vi "Position Space Bar Key.vi"(8 "error in (no error)":errorcluster, 10 "z Key":refnum<vi>, 11 "Space bar Key":refnum<vi>) -> (0 "error out":errorcluster)   [LabVIEW 2014]
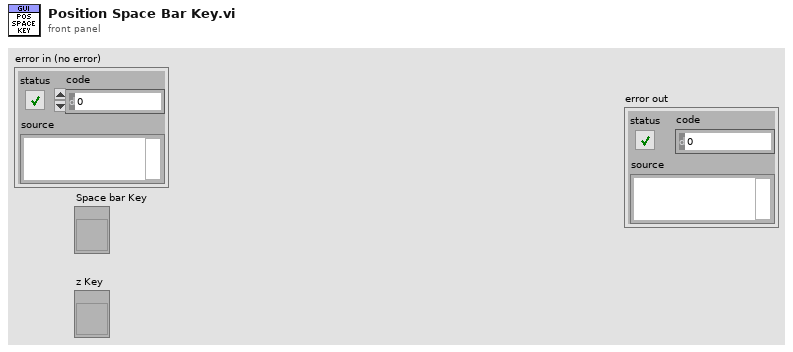
[diagram p1: front panel]
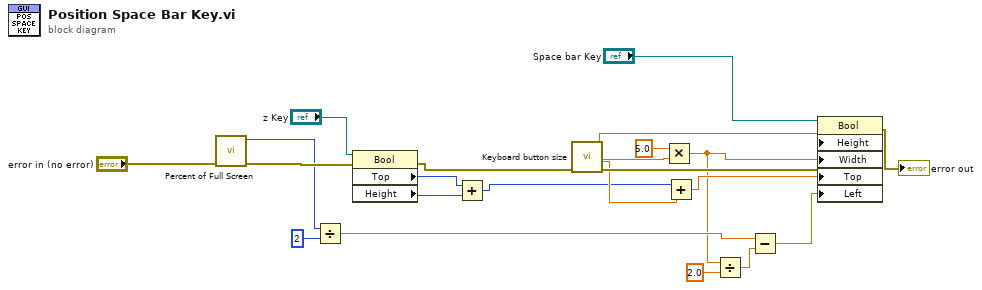
[diagram p0: block diagram]
diagram:
  n1 = call "Percent of Full Screen.vi"("error in (no error)"="error in (no error)") -> ("error out"=w8:errorcluster, "Right"=w7:i16)  [unwired: 8 in, 1 out]
  n2 = Divide(x=w7, y=i16 2) -> (x/y=w5:dbl)
  n3 = property class="Bool"(reference="z Key", error in=w8) -> (error out=w18:errorcluster, "Top"=w16:i32, "Height"=w15:u32)  [unwired: 1 out]
  n4 = Add(x=w16, y=w15) -> (x+y=w13:u32)
  n5 = call "Keyboard button size.vi"("error in (no error)"=w18) -> ("error out"=w21:errorcluster, "Key Spacing"=w14:dbl, "Key Width"=w11:dbl, "Key Height"=w19:dbl)  [unwired: 7 in]
  n6 = Multiply(x=5.0, y=w11) -> (x*y=w4:dbl)
  n7 = Add(x=w13, y=w14) -> (x+y=w12:dbl)
  n8 = Divide(x=w4, y=2.0) -> (x/y=w2:dbl)
  n9 = Subtract(x=w5, y=w2) -> (x-y=w1:dbl)
  n10 = property class="Bool"(reference="Space bar Key", error in=w21, "Height"=w19, "Width"=w4, "Top"=w12, "Left"=w1) -> (error out=→"error out":errorcluster)  [unwired: 1 out]
